vi "display.vi"(0 "raw data":string[](array[string]), 5 "raw data buffer":string[](array[string]), 7 "measurement data":dbl[][](array[numeric]), 9 "buffer plot":cluster{"X":dbl[], "Y":dbl[]}) -> (6 "raw data buffer out":string[](array[string]), 10 "buffer plot out":cluster{"X":dbl[], "Y":dbl[]})   [LabVIEW 2010]
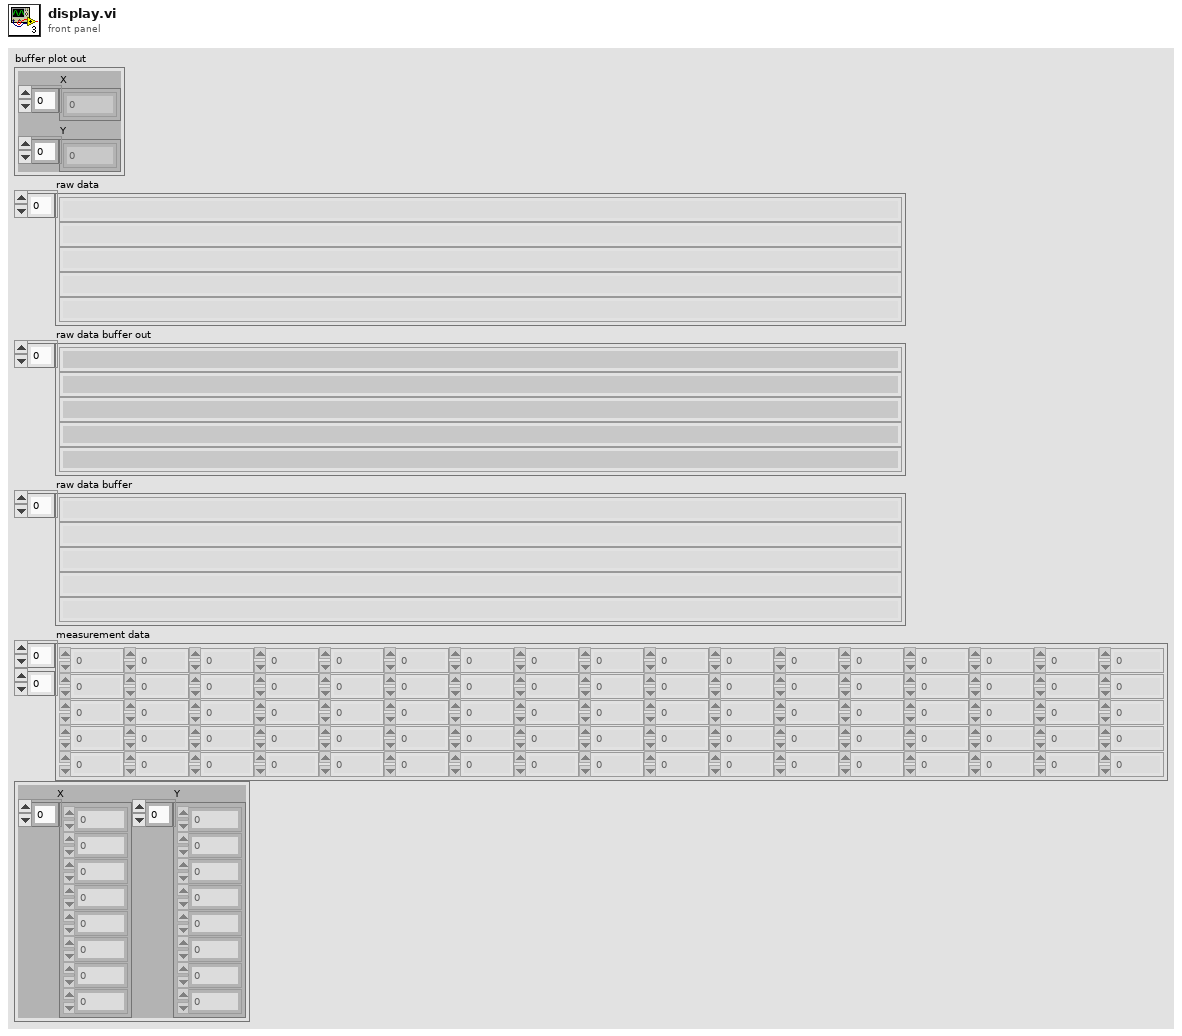
[diagram p1: front panel]
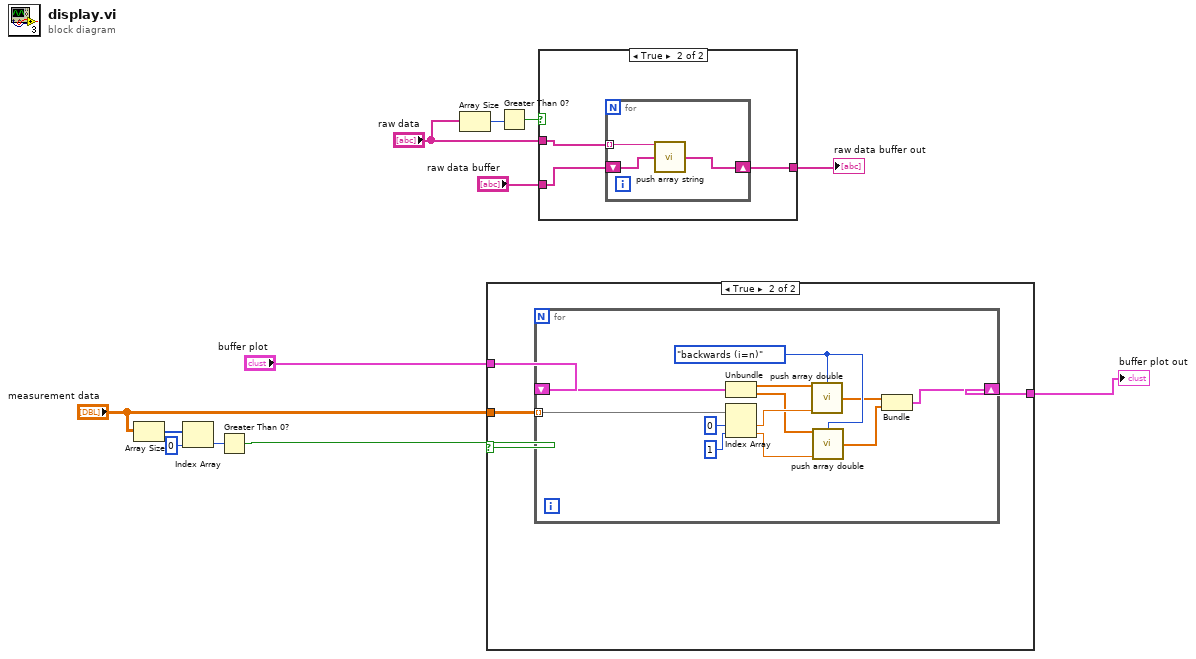
[diagram p0: block diagram]
diagram:
  n1 = Array Size(array="measurement data") -> (size(s)=w6:i32[])
  n2 = Index Array(array=w6, index=0 ("Index")) -> (element=w4:i32)
  n3 = Greater Than 0?(x=w4) -> (x > 0?=w1:bool)
  n4 = Array Size(array="raw data") -> (size(s)=w11:i32)
  n5 = case shown="True" w1 {
    tunnel: "measurement data" -> [_ w16]
    tunnel: "buffer plot" -> [w13 w15]
    tunnel: [w13 w14] -> w2
    frame False {
    }
    frame True {
      n6 = for {
        tunnel: w16 -> [w28] mode=indexing
        shift-right: [w27] -> w14
        shift-left: w15 -> [w26]
        w19 = enum16{"forwards (i=0)", "backwards (i=n)"}."backwards (i=n)" ("mode")
        n7 = Unbundle(w26) -> ("X"=w22:dbl[], "Y"=w21:dbl[])
        n8 = Index Array(array=w28, index #1=0 ("Index"), index #2=1 ("Index")) -> (element #1=w25:dbl, element #2=w20:dbl)
        n9 = call "push array double.vi"("Array"=w22, "mode"=w19, "Element"=w25) -> ("Array out"=w18:dbl[])  [unwired: 12 in]
        n10 = call "push array double.vi"("Array"=w21, "mode"=w19, "Element"=w20) -> ("Array out"=w17:dbl[])  [unwired: 12 in]
        n11 = Bundle("Array out"=w18, "Array out"=w17) -> (w27:cluster{"Array out":dbl[], "Array out":dbl[]})  [unwired: 1 in]
      }
    }
  }
  "buffer plot out" <- w2
  n12 = Greater Than 0?(x=w11) -> (x > 0?=w10:bool)
  n13 = case shown="True" w10 {
    tunnel: "raw data" -> [_ w30]
    tunnel: [w29 w32] -> w7
    tunnel: "raw data buffer" -> [w29 w31]
    frame False {
    }
    frame True {
      n14 = for {
        shift-right: [w35] -> w32
        shift-left: w31 -> [w34]
        tunnel: w30 -> [w33] mode=indexing
        n15 = call "push array string.vi"("Element"=w33, "Array"=w34) -> ("Array out"=w35:string[])  [unwired: 13 in]
      }
    }
  }
  "raw data buffer out" <- w7
